vi "Handle error.vi"(8 "error in (no error)":errorcluster, 11 "RxTx in":refnum<class "RxTx.lvclass">) -> (0 "error out":errorcluster, 3 "RxTx out":refnum<class "RxTx.lvclass">)   [LabVIEW 2018, in "RxTx.lvclass"]
uses:
  RxTx.lvclass
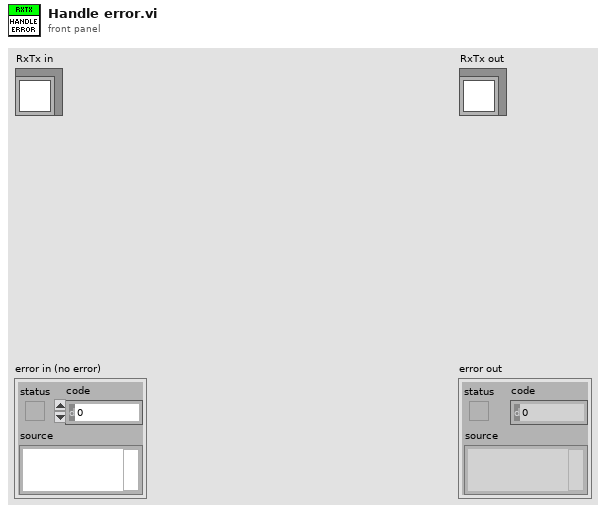
[diagram p1: front panel]
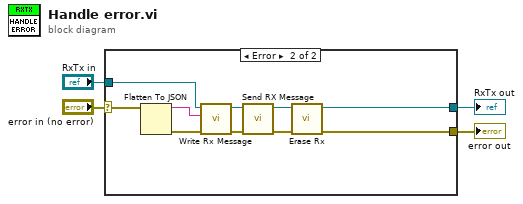
[diagram p0: block diagram]
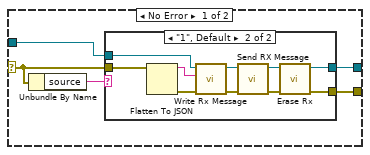
[diagram p2: hidden frame]
diagram:
  n1 = case shown="Error" "error in (no error)" {
    selector: "error in (no error)" -> [w6 w31]
    tunnel: [w7 w27] -> w3
    tunnel: [w8 w26] -> w1
    tunnel: "RxTx in" -> [w9 w23]
    frame No Error {
      n2 = Unbundle By Name(w6) -> ("source"=w5:string)
      n3 = case shown="\"1\", Default" w5 {
        tunnel: w9 -> [w11 w14]
        tunnel: [w11 w20] -> w8
        tunnel: w6 -> [w10 w21]
        tunnel: [w10 w19] -> w7
        frame "" {
        }
        frame "1", Default {
          n4 = Flatten To JSON(anything=w21) -> (JSON string=w15:string, 11:w16:errorcluster)  [unwired: 2 in]
          n5 = call "Write Rx Message.vi"("error in (no error)"=w16, "Rx Message"=w15, "RxTx in"=w14) -> ("error out"=w17:errorcluster, "RxTx out"=w13:refnum<class "RxTx.lvclass">)  [unwired: 7 in]
          n6 = call "Send RX Message.vi"("error in (no error)"=w17, "RxTx in"=w13) -> ("error out"=w18:errorcluster, "RxTx out"=w12:refnum<class "RxTx.lvclass">)  [unwired: 8 in]
          n7 = call "Erase Rx.vi"("error in (no error)"=w18, "RxTx in"=w12) -> ("error out"=w19:errorcluster, "RxTx out"=w20:refnum<class "RxTx.lvclass">)  [unwired: 8 in]
        }
      }
    }
    frame Error {
      n8 = Flatten To JSON(anything=w31) -> (JSON string=w22:string, 11:w28:errorcluster)  [unwired: 2 in]
      n9 = call "Write Rx Message.vi"("error in (no error)"=w28, "Rx Message"=w22, "RxTx in"=w23) -> ("error out"=w29:errorcluster, "RxTx out"=w24:refnum<class "RxTx.lvclass">)  [unwired: 7 in]
      n10 = call "Send RX Message.vi"("error in (no error)"=w29, "RxTx in"=w24) -> ("error out"=w30:errorcluster, "RxTx out"=w25:refnum<class "RxTx.lvclass">)  [unwired: 8 in]
      n11 = call "Erase Rx.vi"("error in (no error)"=w30, "RxTx in"=w25) -> ("error out"=w27:errorcluster, "RxTx out"=w26:refnum<class "RxTx.lvclass">)  [unwired: 8 in]
    }
  }
  "error out" <- w3
  "RxTx out" <- w1
